vi "Swap Floating Point.vi"(5 "DBL Data":dbl[](array[numeric])) -> (2 "Swapped SGL Data":sgl[](array[numeric]))   [LabVIEW 2018]
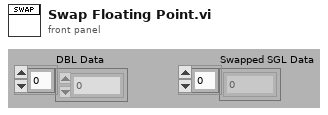
[diagram p1: front panel]
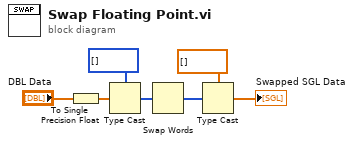
[diagram p0: block diagram]
diagram:
  n1 = To Single Precision Float(number="DBL Data") -> (single precision float=w1:sgl[])
  n2 = Type Cast(type=u32[] [], x=w1) -> (*(type *) &x=w3:u32[])
  n3 = Swap Words(1:w3) -> (0:w4:u32[])
  n4 = Type Cast(type=sgl[] [], x=w4) -> (*(type *) &x=→"Swapped SGL Data":sgl[])
